vi "tempertarue.vi"() -> ()   [LabVIEW 2018]
panel:
  out "output":dbl
  in  "y":dbl
  in  "x":dbl
  in  "?":u8
  out "F 2":dbl(slide) scale=0.0..500.0
  out "F":dbl(slide) scale=0.0..1000.0
  in  "C":dbl
  # "C2"
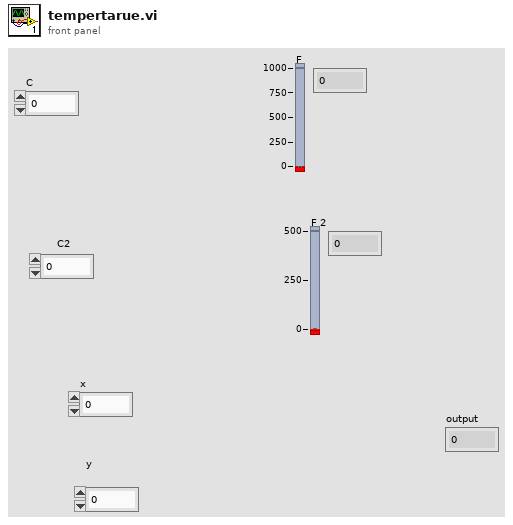
[diagram p1: front panel]
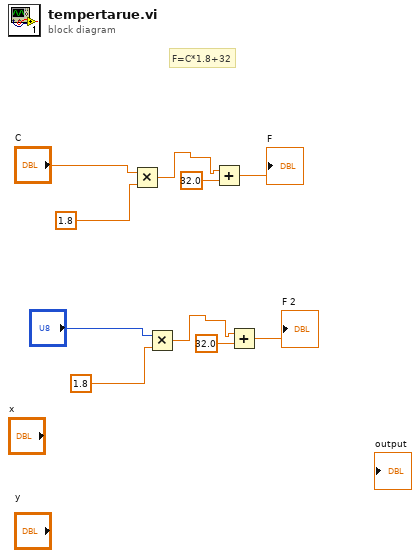
[diagram p0: block diagram]
diagram:
  # "F=C*1.8+32"
  n1 = Multiply(x="C", y=1.8) -> (x*y=w7:dbl)
  n2 = Multiply(x="?", y=1.8) -> (x*y=w4:dbl)
  n3 = Add(x=w7, y=32.0) -> (x+y=→"F":dbl)
  n4 = Add(x=w4, y=32.0) -> (x+y=→"F 2":dbl)
